vi "interp_2d.vi"(10 "z":dbl[](array[numeric]), 11 "prelookup":cluster{"frac":dbl, "num":u8}) -> (3 "z":dbl)   [LabVIEW 2014]
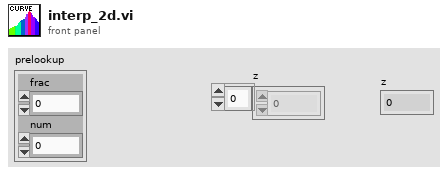
[diagram p1: front panel]
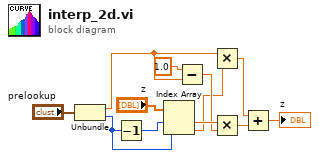
[diagram p0: block diagram]
diagram:
  n1 = Unbundle("prelookup") -> ("frac"=w9:dbl, "num"=w4:u8)
  n2 = Decrement(x=w4) -> (x-1=w5:u8)
  n3 = Index Array(array="z", index #1=w5, index #2=w4) -> (element #1=w3:dbl, element #2=w1:dbl)
  n4 = Subtract(x=1.0, y=w9) -> (x-y=w2:dbl)
  n5 = Multiply(x=w9, y=w1) -> (x*y=w8:dbl)
  n6 = Multiply(x=w3, y=w2) -> (x*y=w7:dbl)
  n7 = Add(x=w8, y=w7) -> (x+y=→"z":dbl)
